vi "clearDisplay.vi"(8 "error in (no error)":errorcluster, 11 "ScriptEditorV2 in":refnum<class "ScriptEditorV2.lvclass">) -> (0 "error out":errorcluster, 3 "ScriptEditorV2 out":refnum<class "ScriptEditorV2.lvclass">)   [LabVIEW 2011, in "Views.lvlib" / "ScriptEditor.lvlib" / "ScriptEditorV2.lvclass"]
uses:
  ScriptEditorV2.lvclass
  ScriptEditorV2.lvclass/ScriptEditorV2.ctl
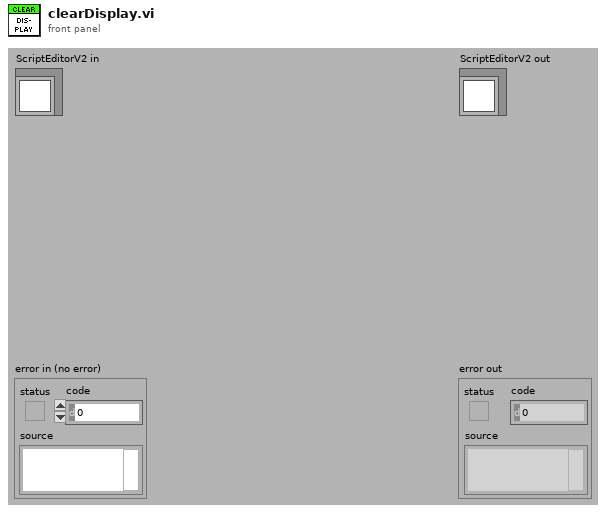
[diagram p1: front panel]
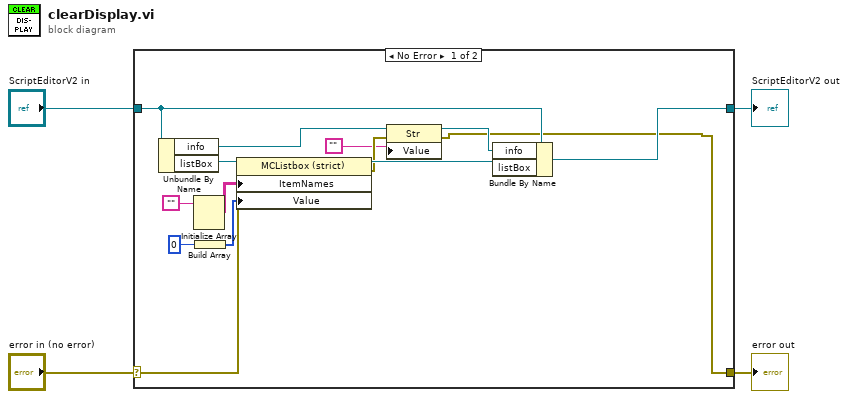
[diagram p0: block diagram]
diagram:
  n1 = case shown="No Error" "error in (no error)" {
    selector: "error in (no error)" -> [w11 w20]
    tunnel: [w5 w20] -> w3
    tunnel: [w6 w19] -> w1
    tunnel: "ScriptEditorV2 in" -> [w12 w19]
    frame No Error {
      n2 = Unbundle By Name(w12) -> ("info"=w9:refnum<vi>, "listBox"=w18:refnum<vi>)
      n3 = Initialize Array("") -> (w17:string[][])  [unwired: 2 in]
      n4 = Build Array(0) -> (w14:i32[])
      n5 = property class="MCListbox (strict)"(reference=w18, error in=w11, "ItemNames"=w17, "Value"=w14) -> (reference out=w13:refnum<vi>, error out=w10:errorcluster)
      n6 = property class="Str"(reference=w9, error in=w10, "Value"="") -> (reference out=w7:refnum<vi>, error out=w5:errorcluster)
      n7 = Bundle By Name(cluster=w12, "info"=w7, "listBox"=w13) -> (w6:refnum<class "ScriptEditorV2.lvclass">)
    }
    frame Error {
    }
  }
  "error out" <- w3
  "ScriptEditorV2 out" <- w1
